vi "AM Calculate Polynomial Coef.vi"(9 "polynomial order":i32, 10 "Longest Temp Vector":dbl[](array[numeric]), 11 "normalized SG Data":dbl[](array[numeric])) -> (1 "Polynomial Coefficients":dbl[](array[numeric]), 2 "R-square":dbl, 3 "Polynomial Coefficients Str":string)   [LabVIEW 2020, in "Test Driver.lvlib"]
uses:
  Test Driver.lvlib
  <vilib>/Analysis/NI_AALPro.lvlib
  <vilib>/Analysis/6fits.llb/Curve Fitting Criteria.ctl
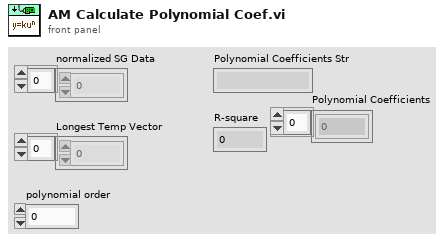
[diagram p1: front panel]
types:
  T1 = typedef "NI_AALPro.lvlib/Curve Fitting Criteria.ctl" = u16
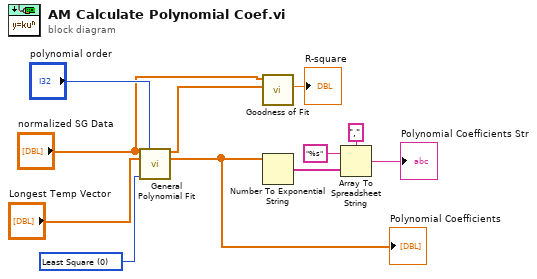
[diagram p0: block diagram]
diagram:
  w9 = T1 0 items=["Least Square", "Least Absolute Residual", "Bisquare"] ("method")
  n1 = call <vilib>:"General Polynomial Fit.vi"("Y"="normalized SG Data", "polynomial order"="polynomial order", "X"="Longest Temp Vector", "method"=w9) -> ("Best Polynomial Fit"=w7:dbl[], "Polynomial Coefficients"=w2:dbl[])  [unwired: 8 in, 2 out]
  "Polynomial Coefficients" <- w2
  n2 = call <vilib>:"Goodness of Fit.vi"("Best Fit"=w7, "Y"="normalized SG Data") -> ("R-square"=→"R-square":dbl)  [unwired: 6 in, 3 out]
  n3 = Number To Exponential String(number=w2) -> (E-format string=w6:string[])  [unwired: 3 in]
  n4 = Array To Spreadsheet String(delimiter (Tab)=",", array=w6, 3:"%s" ("format string")) -> (spreadsheet string=→"Polynomial Coefficients Str":string)
